vi "Relatório.vi"(1 "Resultados médios":string[][](array[string]), 2 "Nome do ensaio":string, 3 "Tabela de resultados":string[][](array[string]), 4 "Círculo de Mohr":cluster{"Array":dbl[], "Array":dbl[]}[][](array[cluster]), 5 "Dados":dbl[][](array[numeric])) -> (0 "error out":errorcluster)   [LabVIEW 2013]
uses:
  <vilib>/Utility/NIReport.llb/NI_report.lvclass
  <vilib>/addons/_office/NI_ReportGenerationToolkit.lvlib
  <vilib>/addons/_office/excel.llb/Excel Easy Table (str).vi
  <vilib>/Utility/NIReport.llb/Excel/NI_Excel.lvclass
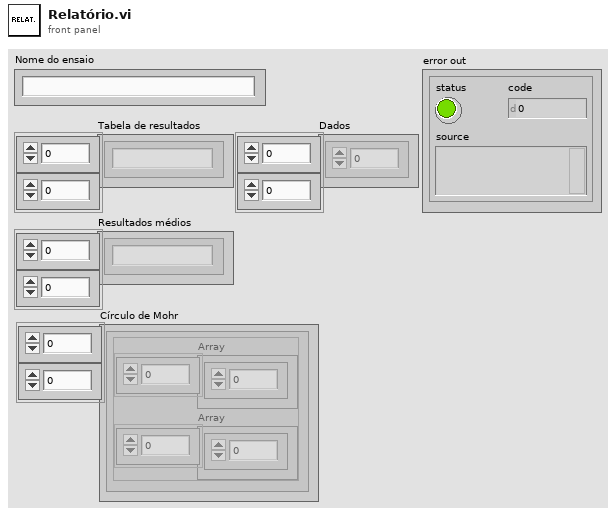
[diagram p1: front panel]
types:
  T1 = cluster{"font style":string, "bold":bool, "italic":bool, "underline":bool, "size":sgl, "color":u32}
  T2 = cluster{"left":i32, "top":i32, "height":dbl, "width":dbl}
  T3 = enum16{"Standard Report", "HTML", "Word", "Excel"}
  T4 = cluster{"Boolean":bool, "Numeric Control":dbl, "Numeric Control":dbl, "scale type":i32}
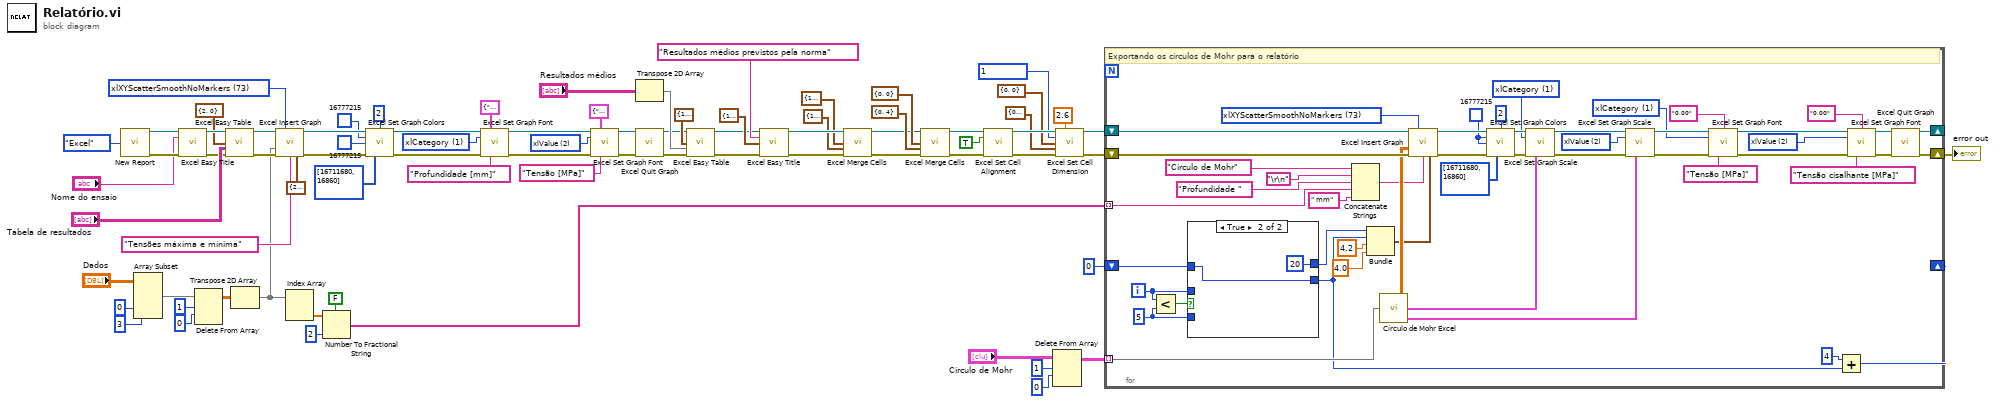
[diagram p0: block diagram]
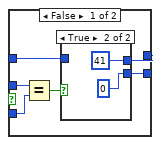
[diagram p2: hidden frame]
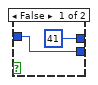
[diagram p3: hidden frame]
diagram:
  w22 = 2 items=["xlCategory"=1, "xlSeriesAxis"=3, "xlValue"=2] ("axis type (xlCategory)")
  w23 = 1 items=["xlCategory"=1, "xlSeriesAxis"=3, "xlValue"=2] ("axis type (xlCategory)")
  w66 = 73 items=["xlColumnClustered"=51, "xlColumnStacked"=52, "xlColumnStacked100"=53, "xl3DColumnClustered"=54, "xl3DColumnStacked"=55, "xl3DColumnStacked100"=56, "xlBarClustered"=57, "xlBarStacked"=58, "xlBarStacked100"=59, "xl3DBarClustered"=60, "xl3DBarStacked"=61, "xl3DBarStacked100"=62, "xlLineStacked"=63, "xlLineStacked100"=64, "xlLineMarkers"=65, "xlLineMarkersStacked"=66, "xlLineMarkersStacked100"=67, "xlPieOfPie"=68, "xlPieExploded"=69, "xl3DPieExploded"=70, "xlBarOfPie"=71, "xlXYScatterSmooth"=72, "xlXYScatterSmoothNoMarkers"=73, "xlXYScatterLines"=74, "xlXYScatterLinesNoMarkers"=75, "xlAreaStacked"=76, "xlAreaStacked100"=77, "xl3DAreaStacked"=78, "xl3DAreaStacked100"=79, "xlDoughnutExploded"=80, "xlRadarMarkers"=81, "xlRadarFilled"=82, "xlSurface"=83, "xlSurfaceWireframe"=84, "xlSurfaceTopView"=85, "xlSurfaceTopViewWireframe"=86, "xlBubble"=15, "xlBubble3DEffect"=87, "xlStockHLC"=88, "xlStockOHLC"=89, "xlStockVHLC"=90, "xlStockVOHLC"=91, "xlCylinderColClustered"=92, "xlCylinderColStacked"=93, "xlCylinderColStacked100"=94, "xlCylinderBarClustered"=95, "xlCylinderBarStacked"=96, "xlCylinderBarStacked100"=97, "xlCylinderCol"=98, "xlConeColClustered"=99, "xlConeColStacked"=100, "xlConeColStacked100"=101, "xlConeBarClustered"=102, "xlConeBarStacked"=103, "xlConeBarStacked100"=104, "xlConeCol"=105, "xlPyramidColClustered"=106, "xlPyramidColStacked"=107, "xlPyramidColStacked100"=108, "xlPyramidBarClustered"=109, "xlPyramidBarStacked"=110, "xlPyramidBarStacked100"=111, "xlPyramidCol"=112, "xl3DColumn"=-4100, "xlLine"=4, "xl3DLine"=-4101, "xl3DPie"=-4102, "xlPie"=5, "xlXYScatter"=-4169, "xl3DArea"=-4098, "xlArea"=1, "xlDoughnut"=-4120, "xlRadar"=-4151] ("graph type (col clustered)")
  n1 = call <vilib>:"New Report.vi"("report type"=T3."Excel") -> ("report out"=w70:refnum<class "NI_report.lvclass">, "error out"=w71:errorcluster)  [unwired: 13 in]
  n2 = Array Subset(array="Dados", index (col)=0 ("index"), length (col)=3 ("length")) -> (w10:dbl[][])  [unwired: 2 in]
  n3 = call <vilib>:"Excel Easy Title.vi"("report in"=w70, "title"="Nome do ensaio", "error in (no error)"=w71) -> ("report out"=w72:refnum<class "NI_report.lvclass">, "error out"=w73:errorcluster)  [unwired: 10 in, 1 out]
  n4 = Delete From Array(array=w10, length=1, index (row)=0) -> (array with subset deleted=w3:dbl[][])  [unwired: 1 in, 1 out]
  n5 = call-poly <vilib>:"Excel Easy Table.vi"("report in"=w72, "start (0, 0)"=cluster{"row":i32, "column":i32} {"row"=2, "column"=0}, "text data"="Tabela de resultados", "error in (no error)"=w73) -> ("report out"=w50:refnum<class "NI_report.lvclass">, "error out"=w49:errorcluster)  [unwired: 7 in, 3 out]
  n6 = Transpose 2D Array(2D array=w3) -> (transposed array=w2:dbl[][])
  n7 = call <vilib>:"Excel Insert Graph.vi"("report in"=w50, "graph type (col clustered)"=w66, "data"=w2, "error in (no error)"=w49, "graph title (\"\")"="Tensões máxima e mínima" ("name (\"\")"), "position/size"=T2 {"left"=2, "top"=8, "height"=4.0, "width"=6.0}) -> ("report out"=w63:refnum<class "NI_report.lvclass">, "error out"=w62:errorcluster)  [unwired: 8 in]
  n8 = Index Array(array=w2) -> (element=w7:dbl[])  [unwired: 2 in]
  n9 = Number To Fractional String(use system decimal point (T)=FALSE, number=w7, precision (6)=i16 2) -> (F-format string=w4:string[])  [unwired: 1 in]
  n10 = call <vilib>:"Excel Set Graph Colors.vi"("report in"=w63, "weight (1)"=i16 2, "graph area color (w)"=u32 16777215, "plot area color (w)"=u32 16777215, "error in (no error)"=w62, "plot colors"=u32[] [16711680, 16860]) -> ("report out"=w25:refnum<class "NI_report.lvclass">, "error out"=w24:errorcluster)  [unwired: 8 in]
  n11 = call <vilib>:"Excel Set Graph Font.vi"("report in"=w25, "axis font"=T1 {"font style"="", "bold"=FALSE, "italic"=FALSE, "underline"=FALSE, "size"=15.0, "color"=4278190080}, "axis type (xlCategory)"=w23, "error in (no error)"=w24, "title (\"\")"="Profundidade [mm]" ("title (\"\")")) -> ("report out"=w21:refnum<class "NI_report.lvclass">, "error out"=w20:errorcluster)  [unwired: 9 in]
  n12 = call <vilib>:"Excel Set Graph Font.vi"("report in"=w21, "axis font"=T1 {"font style"="", "bold"=FALSE, "italic"=FALSE, "underline"=FALSE, "size"=15.0, "color"=4278190080}, "axis type (xlCategory)"=w22, "error in (no error)"=w20, "title (\"\")"="Tensão [MPa]" ("title (\"\")")) -> ("report out"=w19:refnum<class "NI_report.lvclass">, "error out"=w18:errorcluster)  [unwired: 9 in]
  n13 = Transpose 2D Array(2D array="Resultados médios") -> (transposed array=w77:string[][])
  n14 = call <vilib>:"Excel Quit Graph.vi"("report in"=w19, "error in (no error)"=w18) -> ("report out"=w52:refnum<class "NI_report.lvclass">, "error out"=w51:errorcluster)  [unwired: 12 in]
  n15 = call-poly <vilib>:"Excel Easy Table.vi"("report in"=w52, "start (0, 0)"=cluster{"row":i32, "column":i32} {"row"=17, "column"=0}, "text data"=w77, "error in (no error)"=w51) -> ("report out"=w42:refnum<class "NI_report.lvclass">, "error out"=w41:errorcluster)  [unwired: 7 in, 3 out]
  n16 = call <vilib>:"Excel Easy Title.vi"("report in"=w42, "title"="Resultados médios previstos pela norma", "start (0, 0)"=cluster{"row":i32, "column":i32} {"row"=15, "column"=0}, "error in (no error)"=w41) -> ("report out"=w46:refnum<class "NI_report.lvclass">, "error out"=w45:errorcluster)  [unwired: 9 in, 1 out]
  n17 = call <vilib>:"Excel Merge Cells.vi"("report in"=w46, "start (-1, -1)"=cluster{"row":i32, "column":i32} {"row"=15, "column"=0} ("start (0, 0)"), "end (-1, -1)"=cluster{"row":i32, "column":i32} {"row"=15, "column"=4} ("start (0, 0)"), "error in (no error)"=w45) -> ("report out"=w38:refnum<class "NI_report.lvclass">, "error out"=w37:errorcluster)  [unwired: 10 in]
  n18 = call <vilib>:"Excel Merge Cells.vi"("report in"=w38, "start (-1, -1)"=cluster{"row":i32, "column":i32} {"row"=0, "column"=0} ("start (0, 0)"), "end (-1, -1)"=cluster{"row":i32, "column":i32} {"row"=0, "column"=4} ("start (0, 0)"), "error in (no error)"=w37) -> ("report out"=w36:refnum<class "NI_report.lvclass">, "error out"=w35:errorcluster)  [unwired: 10 in]
  n19 = call <vilib>:"Excel Set Cell Alignment.vi"("report in"=w36, "wrap text? (F)"=TRUE, "error in (no error)"=w35) -> ("report out"=w33:refnum<class "NI_report.lvclass">, "error out"=w32:errorcluster)  [unwired: 11 in]
  n20 = Delete From Array(array="Círculo de Mohr", length=1, index (row)=0) -> (array with subset deleted=w54:cluster{"Array":dbl[], "Array":dbl[]}[][])  [unwired: 1 in, 1 out]
  n21 = call <vilib>:"Excel Set Cell Dimension.vi"("report in"=w33, "width (-1)"=2.6, "measurement system"=u16 1, "start (-1, -1)"=cluster{"row":i32, "column":i32} {"row"=0, "column"=0}, "end (-1, -1)"=cluster{"row":i32, "column":i32} {"row"=0, "column"=50}, "error in (no error)"=w32) -> ("report out"=w28:refnum<class "NI_report.lvclass">, "error out"=w27:errorcluster)  [unwired: 8 in]
  n22 = for {
    tunnel: w54 -> [w126] mode=indexing
    shift-right: [w116] -> _
    shift-left: w28 -> [w121]
    shift-right: [w115] -> w1
    shift-left: w27 -> [w120]
    shift-right: [w113] -> _
    shift-left: 0 -> [w83]
    tunnel: w4 -> [w101] mode=indexing
    i -> [w80]
    w79 = 5 ("x")
    w91 = 2 items=["xlCategory"=1, "xlSeriesAxis"=3, "xlValue"=2] ("axis type (xlCategory)")
    w94 = 1 items=["xlCategory"=1, "xlSeriesAxis"=3, "xlValue"=2] ("axis type (xlCategory)")
    w108 = 2 items=["xlCategory"=1, "xlSeriesAxis"=3, "xlValue"=2] ("axis type (xlCategory)")
    w110 = 1 items=["xlCategory"=1, "xlSeriesAxis"=3, "xlValue"=2] ("axis type (xlCategory)")
    w118 = 73 items=["xlColumnClustered"=51, "xlColumnStacked"=52, "xlColumnStacked100"=53, "xl3DColumnClustered"=54, "xl3DColumnStacked"=55, "xl3DColumnStacked100"=56, "xlBarClustered"=57, "xlBarStacked"=58, "xlBarStacked100"=59, "xl3DBarClustered"=60, "xl3DBarStacked"=61, "xl3DBarStacked100"=62, "xlLineStacked"=63, "xlLineStacked100"=64, "xlLineMarkers"=65, "xlLineMarkersStacked"=66, "xlLineMarkersStacked100"=67, "xlPieOfPie"=68, "xlPieExploded"=69, "xl3DPieExploded"=70, "xlBarOfPie"=71, "xlXYScatterSmooth"=72, "xlXYScatterSmoothNoMarkers"=73, "xlXYScatterLines"=74, "xlXYScatterLinesNoMarkers"=75, "xlAreaStacked"=76, "xlAreaStacked100"=77, "xl3DAreaStacked"=78, "xl3DAreaStacked100"=79, "xlDoughnutExploded"=80, "xlRadarMarkers"=81, "xlRadarFilled"=82, "xlSurface"=83, "xlSurfaceWireframe"=84, "xlSurfaceTopView"=85, "xlSurfaceTopViewWireframe"=86, "xlBubble"=15, "xlBubble3DEffect"=87, "xlStockHLC"=88, "xlStockOHLC"=89, "xlStockVHLC"=90, "xlStockVOHLC"=91, "xlCylinderColClustered"=92, "xlCylinderColStacked"=93, "xlCylinderColStacked100"=94, "xlCylinderBarClustered"=95, "xlCylinderBarStacked"=96, "xlCylinderBarStacked100"=97, "xlCylinderCol"=98, "xlConeColClustered"=99, "xlConeColStacked"=100, "xlConeColStacked100"=101, "xlConeBarClustered"=102, "xlConeBarStacked"=103, "xlConeBarStacked100"=104, "xlConeCol"=105, "xlPyramidColClustered"=106, "xlPyramidColStacked"=107, "xlPyramidColStacked100"=108, "xlPyramidBarClustered"=109, "xlPyramidBarStacked"=110, "xlPyramidBarStacked100"=111, "xlPyramidCol"=112, "xl3DColumn"=-4100, "xlLine"=4, "xl3DLine"=-4101, "xl3DPie"=-4102, "xlPie"=5, "xlXYScatter"=-4169, "xl3DArea"=-4098, "xlArea"=1, "xlDoughnut"=-4120, "xlRadar"=-4151] ("graph type (col clustered)")
    w78 = u32 16777215 ("graph area color (w)")
    # "Exportando os círculos de Mohr para o relatório"
    n23 = Less?(x=w80, y=w79) -> (x < y?=w84:bool)
    n24 = case shown="True" w84 {
      tunnel: w83 -> [w127 w138]
      tunnel: [w129 w138] -> w82
      tunnel: w80 -> [w132 _]
      tunnel: w79 -> [w131 _]
      tunnel: [w128 20] -> w81
      frame False {
        n25 = Equal?(x=w132, y=w131) -> (x = y?=w130:bool)
        n26 = case shown="True" w130 {
          tunnel: [w134 0] -> w129
          tunnel: [41 41] -> w128
          tunnel: w127 -> [w134 _]
          frame False {
          }
          frame True {
          }
        }
      }
      frame True {
      }
    }
    n27 = Concatenate Strings("Círculo de Mohr" ("name (\"\")"), "\r\n", "Profundidade " ("string"), w101, " mm" ("string")) -> (w99:string)
    n28 = Bundle(w81, w82, 4.2, 4.0) -> (w117:cluster{i32, i32, dbl, dbl})  [unwired: 1 in]
    n29 = call "Círculo de Mohr Excel.vi"("Array in"=w126) -> ("Array out"=w119:dbl[][], "Cluster 2"=w109:T4, "Cluster"=w105:T4)
    n30 = call <vilib>:"Excel Insert Graph.vi"("report in"=w121, "graph type (col clustered)"=w118, "data"=w119, "error in (no error)"=w120, "graph title (\"\")"=w99, "position/size"=w117) -> ("report out"=w122:refnum<class "NI_report.lvclass">, "error out"=w123:errorcluster)  [unwired: 8 in]
    n31 = call <vilib>:"Excel Set Graph Colors.vi"("report in"=w122, "weight (1)"=i16 2, "graph area color (w)"=w78, "plot area color (w)"=w78, "error in (no error)"=w123, "plot colors"=u32[] [16711680, 16860]) -> ("report out"=w112:refnum<class "NI_report.lvclass">, "error out"=w111:errorcluster)  [unwired: 8 in]
    n32 = call <vilib>:"Excel Set Graph Scale.vi"("report in"=w112, "axis type (xlCategory)"=w110, "error in (no error)"=w111, "axis config"=w109) -> ("report out"=w107:refnum<class "NI_report.lvclass">, "error out"=w106:errorcluster)  [unwired: 10 in]
    n33 = call <vilib>:"Excel Set Graph Scale.vi"("report in"=w107, "axis type (xlCategory)"=w108, "error in (no error)"=w106, "axis config"=w105) -> ("report out"=w96:refnum<class "NI_report.lvclass">, "error out"=w95:errorcluster)  [unwired: 10 in]
    n34 = call <vilib>:"Excel Set Graph Font.vi"("report in"=w96, "number format (general)"="0,00", "axis type (xlCategory)"=w94, "error in (no error)"=w95, "title (\"\")"="Tensão [MPa]" ("title (\"\")")) -> ("report out"=w90:refnum<class "NI_report.lvclass">, "error out"=w89:errorcluster)  [unwired: 9 in]
    n35 = Add(x=4, y=w82) -> (x+y=w113:i32)
    n36 = call <vilib>:"Excel Set Graph Font.vi"("report in"=w90, "number format (general)"="0,00", "axis type (xlCategory)"=w91, "error in (no error)"=w89, "title (\"\")"="Tensão cisalhante [MPa]" ("title (\"\")")) -> ("report out"=w88:refnum<class "NI_report.lvclass">, "error out"=w87:errorcluster)  [unwired: 9 in]
    n37 = call <vilib>:"Excel Quit Graph.vi"("report in"=w88, "error in (no error)"=w87) -> ("report out"=w116:refnum<class "NI_report.lvclass">, "error out"=w115:errorcluster)  [unwired: 12 in]
  }
  "error out" <- w1
